vi "OpticsIO (FPGA).vi"() -> ()   [LabVIEW 2012]
uses:
  <vilib>/rvi/eio/common/nirviEmuTemplateMethod_errors.vi
  <vilib>/eio/EIONode/EIONode.xnode
panel:
  in  "stop 473nm laser":bool
  in  "stop photodiodes":bool
  in  "PWM 532nm Laser":T1={"Pulse Length (Ticks)"=20000, "Pulse Period (Ticks)"=40000, "Ao (Int)"=16384, "Seq 1 (High)"=FALSE, "Seq 2 (Low)"=FALSE}
  in  "PWM 473nm Laser":T1={"Pulse Length (Ticks)"=20000, "Pulse Period (Ticks)"=40000, "Ao (Int)"=16384, "Seq 1 (High)"=FALSE, "Seq 2 (Low)"=FALSE}
  in  "stop 532nm laser":bool
  out "532nm Photodiode":i16
  out "473nm Photodiode":i16
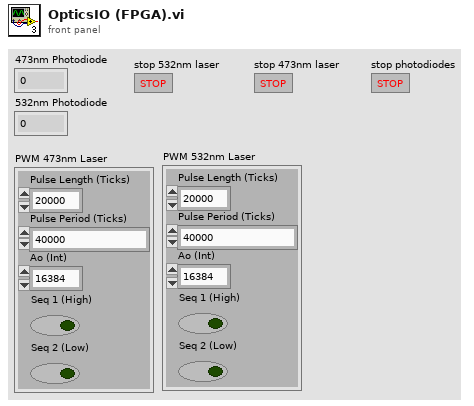
[diagram p1: front panel]
types:
  T1 = cluster{"Pulse Length (Ticks)":u32, "Pulse Period (Ticks)":u32, "Ao (Int)":i32, "Seq 1 (High)":bool, "Seq 2 (Low)":bool}
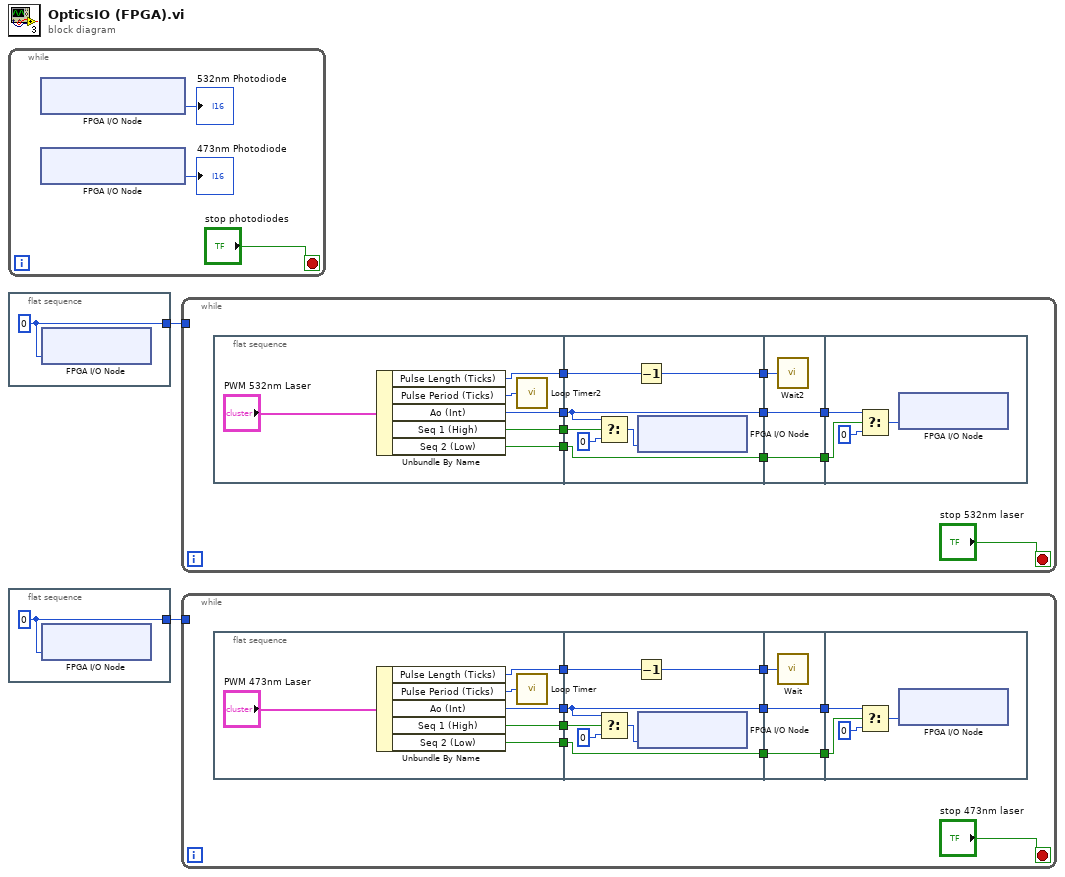
[diagram p0: block diagram]
diagram:
  n1 = while {
    stop <- "stop photodiodes" stop-if-true
    n2 = xnode "FPGA I/O Node"() -> ("532nm Photodiode"=→"532nm Photodiode":i16)  [unwired: 1 in, 1 out]
    n3 = xnode "FPGA I/O Node"() -> ("473nm Photodiode"=→"473nm Photodiode":i16)  [unwired: 1 in, 1 out]
  }
  n4 = flat-sequence {
    tunnel: [w6] -> w2
    frame #0 {
      w6 = i16 0 ("Connector0/AO7")
      n5 = xnode "FPGA I/O Node"("532nm Laser"=w6) -> ()  [unwired: 1 in, 1 out]
    }
  }
  n6 = flat-sequence {
    tunnel: [w7] -> w1
    frame #0 {
      w7 = i16 0 ("Connector0/AO7")
      n7 = xnode "FPGA I/O Node"("473nm Laser"=w7) -> ()  [unwired: 1 in, 1 out]
    }
  }
  n8 = while {
    tunnel: w2 -> [_]
    stop <- "stop 532nm laser" stop-if-true
    n9 = flat-sequence {
      tunnel: [w22] -> w16
      tunnel: [w21] -> w15
      tunnel: [w20] -> w14
      tunnel: [w19] -> w13
      tunnel: [w30] -> w12
      tunnel: w16 -> [w29]
      tunnel: w15 -> [w27]
      tunnel: [w27] -> w11
      tunnel: w14 -> [w26]
      tunnel: [w25] -> w10
      tunnel: w13 -> [w25]
      tunnel: w12 -> [w31]
      tunnel: [w33] -> w9
      tunnel: w11 -> [w33]
      tunnel: [w32] -> w8
      tunnel: w10 -> [w32]
      tunnel: w9 -> [w36]
      tunnel: w8 -> [w35]
      frame #0 {
        n10 = Unbundle By Name("PWM 532nm Laser") -> ("Pulse Length (Ticks)"=w22:u32, "Pulse Period (Ticks)"=w18:u32, "Ao (Int)"=w21:i32, "Seq 1 (High)"=w20:bool, "Seq 2 (Low)"=w19:bool)
        n11 = call "Loop Timer2"("Count(Ticks)"=w18) -> ()  [unwired: 1 out]
      }
      frame #1 {
        n12 = Select(t=w27, s=w26, f=0) -> (s? t:f=w24:i32)
        n13 = Decrement(x=w29) -> (x-1=w30:u32)
        n14 = xnode "FPGA I/O Node"("532nm Laser"=w24) -> ()  [unwired: 1 in, 1 out]
      }
      frame #2 {
        n15 = call "Wait2"("Count(Ticks)"=w31) -> ()  [unwired: 1 out]
      }
      frame #3 {
        n16 = Select(t=w36, s=w35, f=0) -> (s? t:f=w34:i32)
        n17 = xnode "FPGA I/O Node"("532nm Laser"=w34) -> ()  [unwired: 1 in, 1 out]
      }
    }
  }
  n18 = while {
    tunnel: w1 -> [_]
    stop <- "stop 473nm laser" stop-if-true
    n19 = flat-sequence {
      tunnel: [w52] -> w47
      tunnel: [w51] -> w46
      tunnel: [w50] -> w45
      tunnel: [w49] -> w44
      tunnel: [w60] -> w43
      tunnel: w47 -> [w59]
      tunnel: w46 -> [w57]
      tunnel: [w57] -> w42
      tunnel: w45 -> [w56]
      tunnel: [w55] -> w41
      tunnel: w44 -> [w55]
      tunnel: w43 -> [w61]
      tunnel: [w63] -> w40
      tunnel: w42 -> [w63]
      tunnel: [w62] -> w39
      tunnel: w41 -> [w62]
      tunnel: w40 -> [w66]
      tunnel: w39 -> [w65]
      frame #0 {
        n20 = Unbundle By Name("PWM 473nm Laser") -> ("Pulse Length (Ticks)"=w52:u32, "Pulse Period (Ticks)"=w48:u32, "Ao (Int)"=w51:i32, "Seq 1 (High)"=w50:bool, "Seq 2 (Low)"=w49:bool)
        n21 = call "Loop Timer"("Count(Ticks)"=w48) -> ()  [unwired: 1 out]
      }
      frame #1 {
        n22 = Select(t=w57, s=w56, f=0) -> (s? t:f=w54:i32)
        n23 = Decrement(x=w59) -> (x-1=w60:u32)
        n24 = xnode "FPGA I/O Node"("473nm Laser"=w54) -> ()  [unwired: 1 in, 1 out]
      }
      frame #2 {
        n25 = call "Wait"("Count(Ticks)"=w61) -> ()  [unwired: 1 out]
      }
      frame #3 {
        n26 = Select(t=w66, s=w65, f=0) -> (s? t:f=w64:i32)
        n27 = xnode "FPGA I/O Node"("473nm Laser"=w64) -> ()  [unwired: 1 in, 1 out]
      }
    }
  }
